vi "Get Foreign Key.vi"(8 "error in (no error)":errorcluster, 9 "Column Name Array":string[](array[string]), 10 "Table Name":string, 11 "MS Access in":refnum<class "MS Access.lvclass">) -> (0 "error out":errorcluster, 2 "Foreign Key Array":T1(array[cluster]), 3 "MS Access out":refnum<class "MS Access.lvclass">)   [LabVIEW 2020, in "MS Access.lvclass"]
uses:
  MS Access.lvclass
  ODBC/ADODB.lvclass
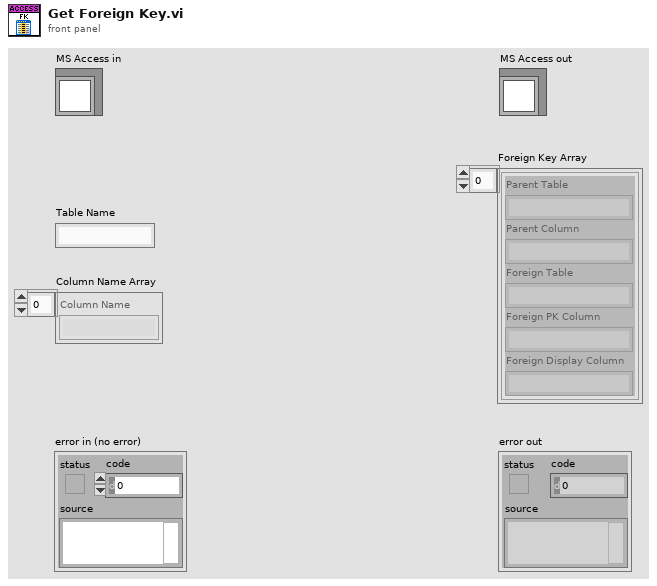
[diagram p1: front panel]
types:
  T1 = cluster{"Parent Table":string, "Parent Column":string, "Foreign Table":string, "Foreign PK Column":string, "Foreign Display Column":string}[]
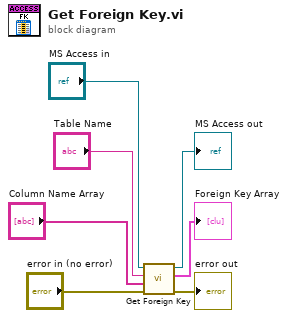
[diagram p0: block diagram]
diagram:
  n1 = call-parent "Get Foreign Key.vi"("error in (no error)"="error in (no error)", "Column Name Array"="Column Name Array", "Table Name"="Table Name", "ADODB in"="MS Access in") -> ("error out"=→"error out":errorcluster, "Foreign Key Array"=→"Foreign Key Array":T1, "ADODB out"=→"MS Access out":refnum<class "MS Access.lvclass">)  [unwired: 5 in]
